vi "Cage controller.vi"(7 "Set/Get":T2, 8 "error in (no error)":errorcluster, 9 "Cluster In":T3, 10 "Action":T1, 11 "reference in":refnum<k24>) -> (0 "error out":errorcluster, 1 "Cluster out":T3, 3 "reference out":refnum<k24>)   [LabVIEW 2018]
uses:
  Thorlabs Translation Stages/Controls/Translation Stage Cluster.ctl
  General/Controls/Translation Stage Types.ctl
  General/Controls/Set Get Controls.ctl
  C:/Project/SSOCT/Labview Software/Thorlabs.MotionControl.Controls.dll
  Thorlabs.MotionControl.Controls.dll
  Thorlabs Translation Stages/Controls/Motion Translation Module Control2.ctl
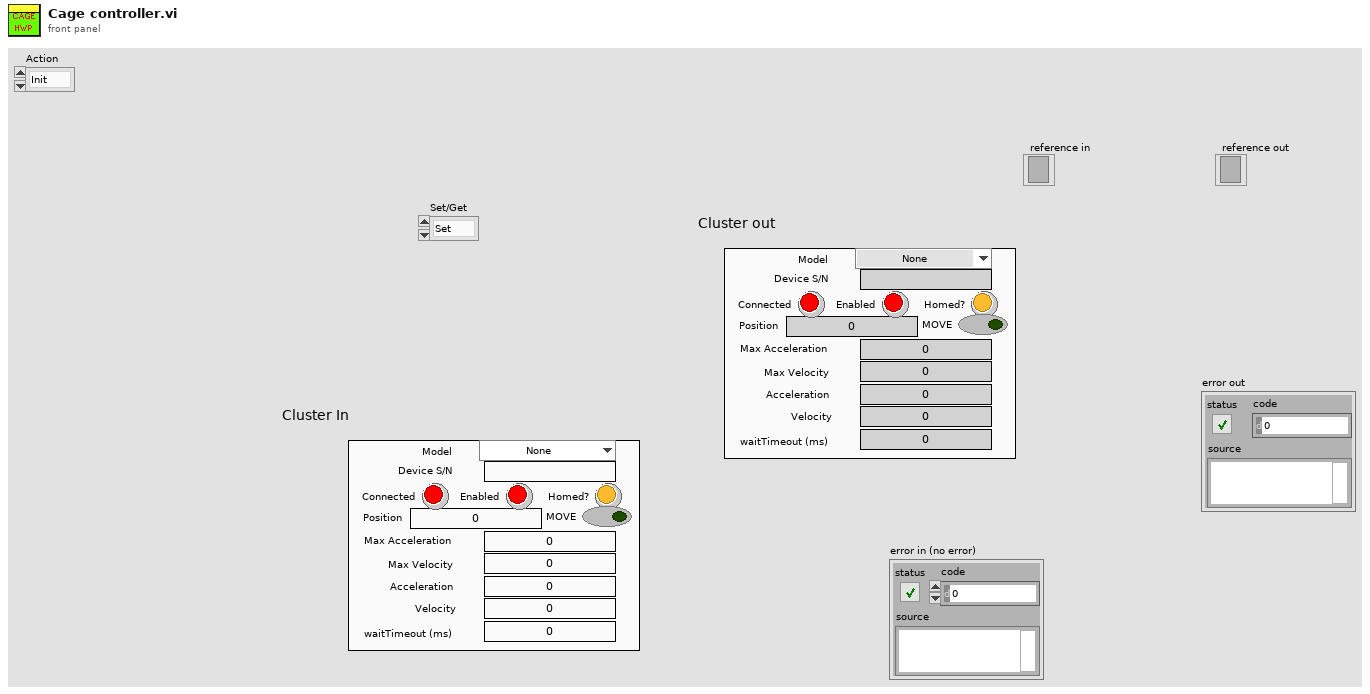
[diagram p1: front panel]
types:
  T1 = typedef "Motion Translation Module Control2.ctl" = enum16{"Init", "Home", "Status", "Velocity/Accel", "Position", "Jog", "Stop", "Uninit", "Enable", "Disable"}
  T2 = typedef "Set Get Controls.ctl" = enum16{"Set", "Get"}
  T3 = typedef "Translation Stage Cluster.ctl" = cluster{"Position":dbl, "Is.Enabled?":bool, "Is.Connected?":bool, "Device SN":string, "AccelerationMaximum":dbl, "VelocityMaximum":dbl, "Acceleration":dbl, "Velocity":dbl, "waitTimeout (ms)":i32, "Model":T4, "Is.Homed?":bool, "MOVE":bool}
  T4 = typedef "Translation Stage Types.ctl" = enum16{"None", "Thorlabs LTS", "Thorlabs MLJ"}
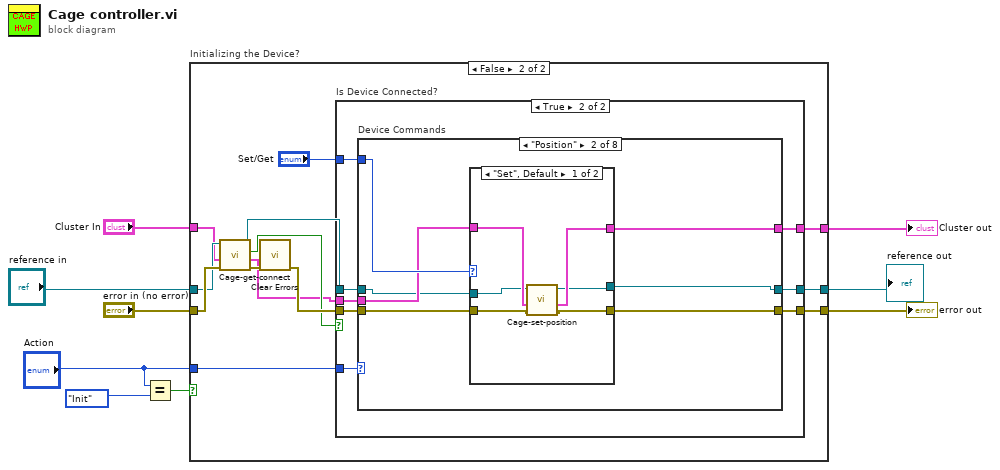
[diagram p0: block diagram]
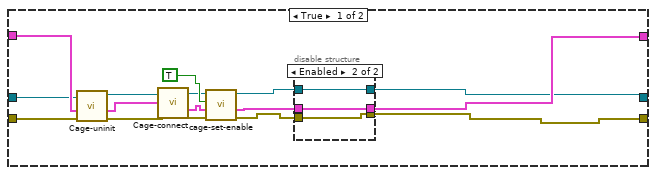
[diagram p2: hidden frame]
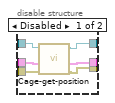
[diagram p3: hidden frame]
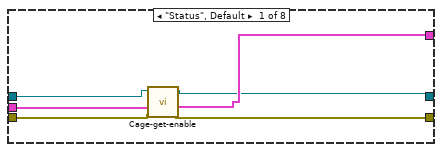
[diagram p5: hidden frame]
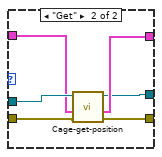
[diagram p6: hidden frame]
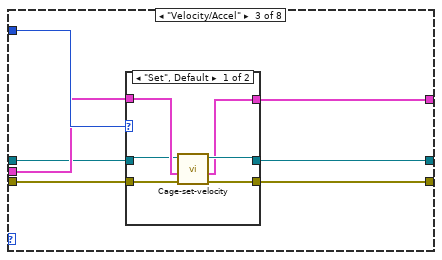
[diagram p7: hidden frame]
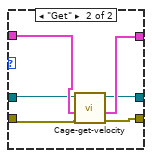
[diagram p8: hidden frame]
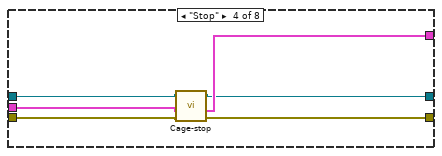
[diagram p9: hidden frame]
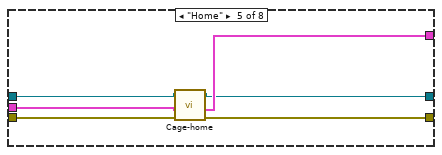
[diagram p10: hidden frame]
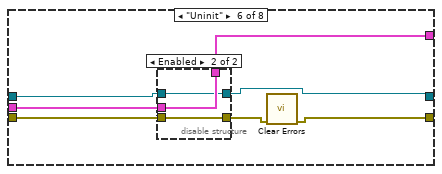
[diagram p11: hidden frame]
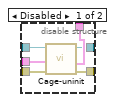
[diagram p12: hidden frame]
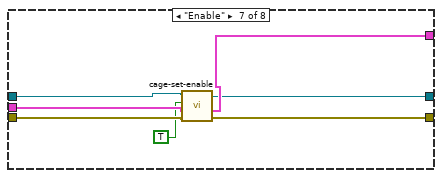
[diagram p13: hidden frame]
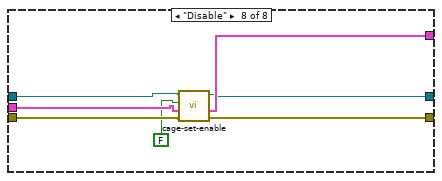
[diagram p14: hidden frame]
diagram:
  n1 = Equal?(x="Action", y=Motion_Translation_Module_Control2."Init" ("Action")) -> (x = y?=w4:bool)
  n2 = case "Initializing the Device?" shown="False" w4 {
    tunnel: "reference in" -> [w11 w39]
    tunnel: [w16 w47] -> w9
    tunnel: [w17 w46] -> w8
    tunnel: [w18 w45] -> w7
    tunnel: "error in (no error)" -> [w15 w40]
    tunnel: "Cluster In" -> [w13 w37]
    tunnel: "Action" -> [_ w44]
    frame True {
      n3 = call "Cage-uninit.vi"("error in (no error)"=w15, "Cluster in"=w13, "reference in"=w11) -> ("error out"=w14:errorcluster, "Cluster out"=w12:T3, "reference out"=w10:refnum<k24>)  [unwired: 5 in, 1 out]
      n4 = call "Cage-connect.vi"("error in (no error)"=w14, "Cluster in"=w12, "reference in"=w10) -> ("error out"=w25:errorcluster, "Cluster out"=w24:T3, "reference out"=w22:refnum<k24>)  [unwired: 5 in, 1 out]
      n5 = call "cage-set-enable.vi"("error in (no error)"=w25, "Cluster in"=w24, "Enable?"=TRUE, "reference in"=w22) -> ("error out"=w21:errorcluster, "Cluster out"=w20:T3, "reference out"=w19:refnum<k24>)  [unwired: 5 in]
      n6 = disable-structure shown="Enabled" {
        disable-tunnel: w21 -> [w31 w32]
        disable-tunnel: w20 -> [w30 w33]
        disable-tunnel: w19 -> [w29 w34]
        disable-tunnel: [w28 w32] -> w18
        disable-tunnel: [w27 w33] -> w17
        disable-tunnel: [w26 w34] -> w16
        frame Disabled {
          n7 = call "Cage-get-position.vi"("error in (no error)"=w31, "Cluster in"=w30, "reference in"=w29) -> ("error out"=w28:errorcluster, "Cluster out"=w27:T3, "reference out"=w26:refnum<k24>)  [unwired: 5 in, 1 out]
        }
        frame Enabled {
        }
      }
    }
    frame False {
      n8 = call "Cage-get-connect.vi"("error in (no error)"=w40, "Cluster in"=w37, "reference in"=w39) -> ("error out"=w41:errorcluster, "Cluster out"=w35:T3, "IsConnected"=w38:bool, "reference out"=w36:refnum<k24>)  [unwired: 5 in]
      n9 = call <vilib>:"Clear Errors.vi"("error in (no error)"=w41) -> ("error out"=w42:errorcluster)  [unwired: 5 in, 1 out]
      n10 = case "Is Device Connected?" shown="True" w38 {
        tunnel: w36 -> [w48 w58]
        tunnel: [w48 w57] -> w47
        tunnel: [w50 w56] -> w46
        tunnel: [w49 w55] -> w45
        tunnel: w42 -> [w49 w54]
        tunnel: "Set/Get" -> [_ w53]
        tunnel: w44 -> [_ w52]
        tunnel: w35 -> [w50 w51]
        frame False {
        }
        frame True {
          n11 = case "Device Commands" shown="\"Position\"" w52 {
            tunnel: w53 -> [_ w71 w90 _ _ _ _ _]
            tunnel: w51 -> [w63 w68 w87 w107 w111 w119 w136 w143]
            tunnel: w54 -> [w64 w70 w89 w108 w114 w120 w137 w144]
            tunnel: [w60 w66 w85 w103 w109 w115 w131 w138] -> w57
            tunnel: [w59 w69 w88 w105 w113 w121 w133 w139] -> w55
            tunnel: [w61 w67 w86 w106 w112 w116 w132 w140] -> w56
            tunnel: w58 -> [w62 w65 w84 w104 w110 w118 w135 w142]
            frame "Status", Default {
              n12 = call "Cage-get-enable.vi"("error in (no error)"=w64, "Cluster in"=w63, "reference in"=w62) -> ("error out"=w59:errorcluster, "Cluster out"=w61:T3, "reference out"=w60:refnum<k24>)  [unwired: 5 in, 1 out]
            }
            frame "Position" {
              n13 = case shown="\"Set\", Default" w71 {
                tunnel: w70 -> [w77 w83]
                tunnel: [w76 w79] -> w69
                tunnel: w68 -> [w74 w81]
                tunnel: [w75 w80] -> w67
                tunnel: w65 -> [w73 w82]
                tunnel: [w72 w78] -> w66
                frame "Set", Default {
                  n14 = call "Cage-set-position.vi"("error in (no error)"=w77, "Cluster in"=w74, "reference in"=w73) -> ("error out"=w76:errorcluster, "Cluster out"=w75:T3, "reference out"=w72:refnum<k24>)  [unwired: 6 in]
                }
                frame "Get" {
                  n15 = call "Cage-get-position.vi"("error in (no error)"=w83, "Cluster in"=w81, "reference in"=w82) -> ("error out"=w79:errorcluster, "Cluster out"=w80:T3, "reference out"=w78:refnum<k24>)  [unwired: 5 in, 1 out]
                }
              }
            }
            frame "Velocity/Accel" {
              n16 = case shown="\"Set\", Default" w90 {
                tunnel: w89 -> [w96 w102]
                tunnel: [w95 w101] -> w88
                tunnel: w87 -> [w92 w100]
                tunnel: [w93 w99] -> w86
                tunnel: w84 -> [w91 w98]
                tunnel: [w94 w97] -> w85
                frame "Set", Default {
                  n17 = call "Cage-set-velocity.vi"("error in (no error)"=w96, "Cluster in"=w92, "reference in"=w91) -> ("error out"=w95:errorcluster, "Cluster out"=w93:T3, "reference out"=w94:refnum<k24>)  [unwired: 5 in, 1 out]
                }
                frame "Get" {
                  n18 = call "Cage-get-velocity.vi"("error in (no error)"=w102, "Cluster in"=w100, "reference in"=w98) -> ("error out"=w101:errorcluster, "Cluster out"=w99:T3, "reference out"=w97:refnum<k24>)  [unwired: 5 in, 1 out]
                }
              }
            }
            frame "Stop" {
              n19 = call "Cage-stop.vi"("error in (no error)"=w108, "Cluster in"=w107, "reference in"=w104) -> ("error out"=w105:errorcluster, "Cluster out"=w106:T3, "reference out"=w103:refnum<k24>)  [unwired: 6 in]
            }
            frame "Home" {
              n20 = call "Cage-home.vi"("error in (no error)"=w114, "Cluster in"=w111, "reference in"=w110) -> ("error out"=w113:errorcluster, "Cluster out"=w112:T3, "reference out"=w109:refnum<k24>)  [unwired: 6 in]
            }
            frame "Uninit" {
              n21 = disable-structure shown="Enabled" {
                disable-tunnel: w120 -> [w127 w128]
                disable-tunnel: w119 -> [w126 w130]
                disable-tunnel: w118 -> [w125 w129]
                disable-tunnel: [w124 w128] -> w117
                disable-tunnel: [w123 w130] -> w116
                disable-tunnel: [w122 w129] -> w115
                frame Disabled {
                  n22 = call "Cage-uninit.vi"("error in (no error)"=w127, "Cluster in"=w126, "reference in"=w125) -> ("error out"=w124:errorcluster, "Cluster out"=w123:T3, "reference out"=w122:refnum<k24>)  [unwired: 5 in, 1 out]
                }
                frame Enabled {
                }
              }
              n23 = call <vilib>:"Clear Errors.vi"("error in (no error)"=w117) -> ("error out"=w121:errorcluster)  [unwired: 5 in, 1 out]
            }
            frame "Enable" {
              n24 = call "cage-set-enable.vi"("error in (no error)"=w137, "Cluster in"=w136, "Enable?"=TRUE, "reference in"=w135) -> ("error out"=w133:errorcluster, "Cluster out"=w132:T3, "reference out"=w131:refnum<k24>)  [unwired: 5 in]
            }
            frame "Disable" {
              n25 = call "cage-set-enable.vi"("error in (no error)"=w144, "Cluster in"=w143, "Enable?"=FALSE, "reference in"=w142) -> ("error out"=w139:errorcluster, "Cluster out"=w140:T3, "reference out"=w138:refnum<k24>)  [unwired: 5 in]
            }
          }
        }
      }
    }
  }
  "Cluster out" <- w8
  "error out" <- w7
  "reference out" <- w9
